vi "EstimateTargetingInformation.vi"(0 "X (in) [t0]":dbl, 5 "Y (in) [t0]":dbl, 7 "Robot Heading (deg)":dbl, 12 "Acceptable Heading Error (deg)":dbl, 13 "Min Timed Aligned (ms)":u32) -> (4 "Pointed At Target":bool, 6 "Heading to Target (deg)":dbl, 8 "Distance to Target (in)":dbl, 15 "Targeting Information":dbl[](array[numeric]))   [LabVIEW 2020]
doc: "This VI estimates the robot's heading and distance to the nearest requested scoring location."
uses:
  <vilib>/Rock Robotics/WPI/DriverStation/WPI_DriverStationAllianceInfo.ctl
  GlobalArm.vi
  GlobalDriverStationData.vi
  GlobalPoseAndTargeting.vi
  GlobalDriverStationCommands.vi
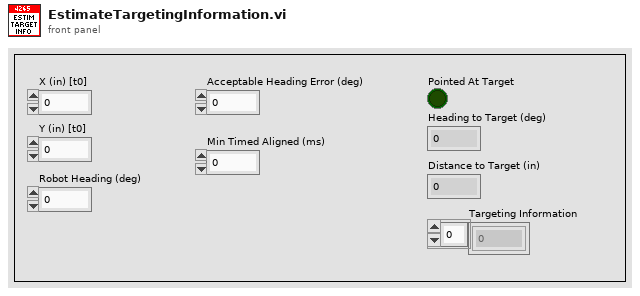
[diagram p1: front panel]
types:
  T1 = typedef "WPI_DriverStationAllianceInfo.ctl" = enum16{"Red", "Blue", "Invalid"}
  T2 = enum16{"Low Cube", "Mid Cube", "High Cube", "Low Cone", "Mid Cone", "High Cone"}
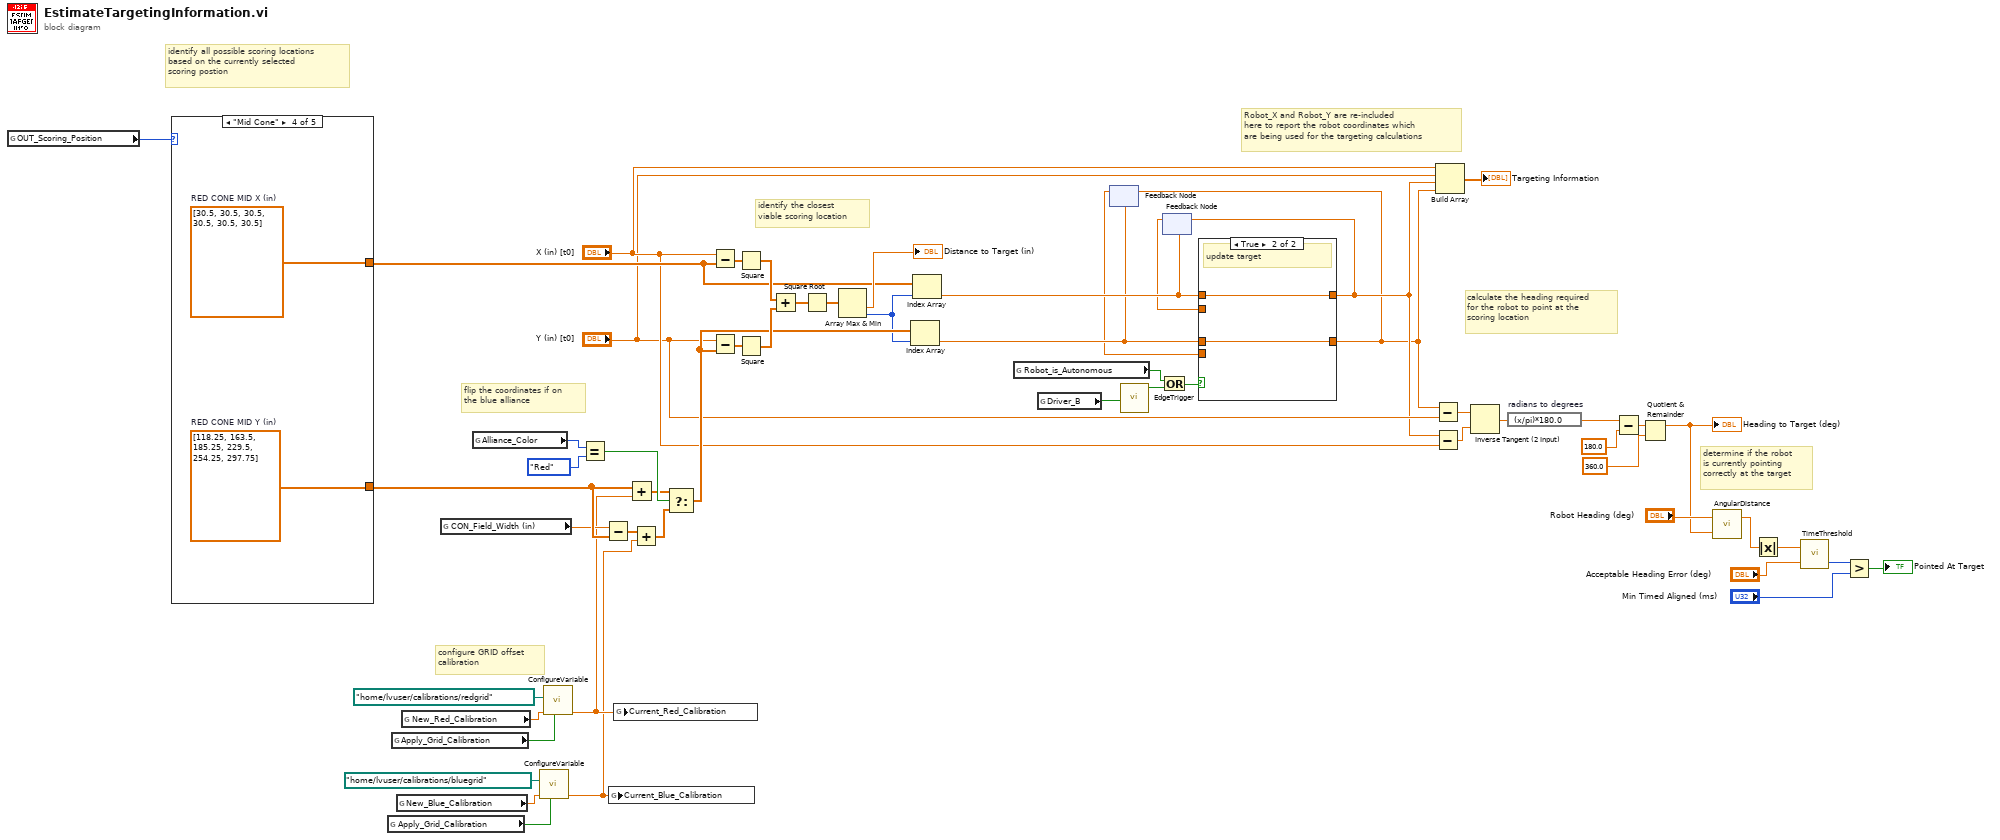
[diagram p0: block diagram]
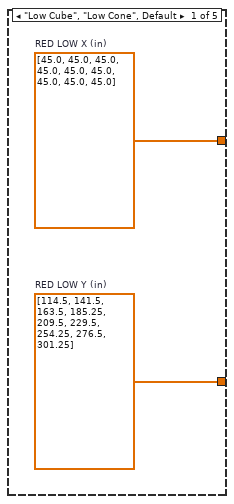
[diagram p3: hidden frame]
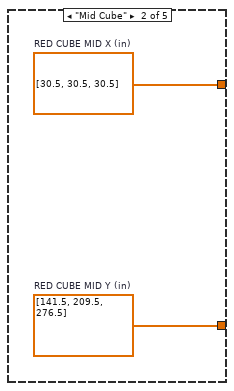
[diagram p4: hidden frame]
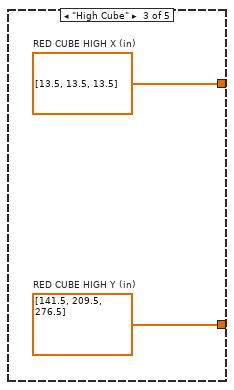
[diagram p5: hidden frame]
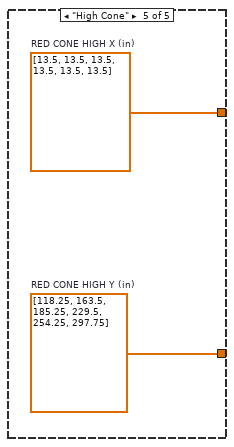
[diagram p6: hidden frame]
diagram:
  # "configure GRID offset\ncalibration"
  # "Robot_X and Robot_Y are re-included\nhere to report the robot coordinates which\nare being used for the targeting calculations"
  # "determine if the robot\nis currently pointing\ncorrectly at the target"
  # "calculate the heading required\nfor the robot to point at the\nscoring location"
  # "identify the closest\nviable scoring location"
  # "flip the coordinates if on\nthe blue alliance"
  # "identify all possible scoring locations\nbased on the currently selected\nscoring postion"
  n1 = global read "GlobalArm.vi" "OUT_Scoring_Position"() -> (w13:T2)
  n2 = case shown="\"Mid Cone\"" w13 {
    tunnel: [w57 w59 w61 w63 w65] -> w41
    tunnel: [w56 w58 w60 w62 w64] -> w51
    frame "Low Cube", "Low Cone", Default {
      w56 = dbl[] [114.5, 141.5, 163.5, 185.25, 209.5, 229.5, 254.25, 276.5, 301.25]  # RED LOW Y (in)
      w57 = dbl[] [45.0, 45.0, 45.0, 45.0, 45.0, 45.0, 45.0, 45.0, 45.0]  # RED LOW X (in)
    }
    frame "Mid Cube" {
      w58 = dbl[] [141.5, 209.5, 276.5]  # RED CUBE MID Y (in)
      w59 = dbl[] [30.5, 30.5, 30.5]  # RED CUBE MID X (in)
    }
    frame "High Cube" {
      w60 = dbl[] [141.5, 209.5, 276.5]  # RED CUBE HIGH Y (in)
      w61 = dbl[] [13.5, 13.5, 13.5]  # RED CUBE HIGH X (in)
    }
    frame "Mid Cone" {
      w62 = dbl[] [118.25, 163.5, 185.25, 229.5, 254.25, 297.75]  # RED CONE MID Y (in)
      w63 = dbl[] [30.5, 30.5, 30.5, 30.5, 30.5, 30.5]  # RED CONE MID X (in)
    }
    frame "High Cone" {
      w64 = dbl[] [118.25, 163.5, 185.25, 229.5, 254.25, 297.75]  # RED CONE HIGH Y (in)
      w65 = dbl[] [13.5, 13.5, 13.5, 13.5, 13.5, 13.5]  # RED CONE HIGH X (in)
    }
  }
  n3 = global read "GlobalPoseAndTargeting.vi" "Apply_Grid_Calibration"() -> (w5:bool)
  n4 = global read "GlobalPoseAndTargeting.vi" "Apply_Grid_Calibration"() -> (w9:bool)
  n5 = global read "GlobalPoseAndTargeting.vi" "New_Blue_Calibration"() -> (w6:dbl)
  n6 = global read "GlobalPoseAndTargeting.vi" "New_Red_Calibration"() -> (w10:dbl)
  n7 = global read "GlobalPoseAndTargeting.vi" "CON_Field_Width (in)"() -> (w49:dbl)
  n8 = global read "GlobalDriverStationData.vi" "Alliance_Color"() -> (w54:T1)
  n9 = call "ConfigureVariable.vi"("Apply New Setpoint"=w5, "New Setpoint Value"=w6, "Setpoint Save Location"=path "/home/lvuser/calibrations/bluegrid") -> ("Selected Setpoint Value"=w4:dbl)  [unwired: 8 in]
  n10 = call "ConfigureVariable.vi"("Apply New Setpoint"=w9, "New Setpoint Value"=w10, "Setpoint Save Location"=path "/home/lvuser/calibrations/redgrid") -> ("Selected Setpoint Value"=w8:dbl)  [unwired: 8 in]
  n11 = Equal?(x=w54, y=WPI_DriverStationAllianceInfo."Red") -> (x = y?=w52:bool)
  n12 = Subtract(x=w49, y=w51) -> (x-y=w50:dbl[])
  n13 = global write "GlobalPoseAndTargeting.vi" "Current_Blue_Calibration"(w4) -> ()
  n14 = global write "GlobalPoseAndTargeting.vi" "Current_Red_Calibration"(w8) -> ()
  n15 = Add(x=w51, y=w8) -> (x+y=w20:dbl[])
  n16 = Add(x=w50, y=w4) -> (x+y=w21:dbl[])
  n17 = Select(t=w20, s=w52, f=w21) -> (s? t:f=w40:dbl[])
  n18 = Subtract(x="X (in) [t0]", y=w41) -> (x-y=w48:dbl[])
  n19 = Subtract(x="Y (in) [t0]", y=w40) -> (x-y=w47:dbl[])
  n20 = Square(x=w48) -> (x^2=w46:dbl[])
  n21 = Square(x=w47) -> (x^2=w45:dbl[])
  n22 = Add(x=w46, y=w45) -> (x+y=w44:dbl[])
  n23 = Square Root(x=w44) -> (sqrt(x)=w43:dbl[])
  n24 = Array Max & Min(array=w43) -> (min value=→"Distance to Target (in)":dbl, min index (indices)=w39:i32)  [unwired: 2 out]
  n25 = Index Array(array=w40, index=w39) -> (element=w16:dbl)
  n26 = Index Array(array=w41, index=w39) -> (element=w18:dbl)
  n27 = global read "GlobalDriverStationData.vi" "Robot_is_Autonomous"() -> (w1:bool)
  n28 = global read "GlobalDriverStationCommands.vi" "Driver_B"() -> (w12:bool)
  n29 = feedback #1(w16) -> (w14:dbl)
  n30 = call "EdgeTrigger.vi"("Input Signal"=w12) -> ("Rising Edge Trigger"=w2:bool)  [unwired: 2 out]
  n31 = Or(x=w1, y=w2) -> (x .or. y?=w3:bool)
  n32 = feedback #2(w18) -> (w17:dbl)
  n33 = case shown="True" w3 {
    tunnel: w18 -> [_ w69]
    tunnel: w16 -> [_ w68]
    tunnel: [w67 w69] -> w19
    tunnel: [w66 w68] -> w15
    tunnel: w17 -> [w67 _]
    tunnel: w14 -> [w66 _]
    frame False {
      # "use latched target"
    }
    frame True {
      # "update target"
    }
  }
  n34 = feedback-in #1(w15) -> ()
  n35 = feedback-in #2(w19) -> ()
  n36 = Subtract(x=w15, y="Y (in) [t0]") -> (x-y=w37:dbl)
  n37 = Subtract(x=w19, y="X (in) [t0]") -> (x-y=w36:dbl)
  n38 = Build Array("X (in) [t0]", "Y (in) [t0]", w19, w15) -> (→"Targeting Information":dbl[])
  n39 = Inverse Tangent (2 Input)(1:w36, 2:w37) -> (0:w38:dbl)
  n40 = expression code="(x/pi)*180.0" "radians to degrees"(w38) -> (w25:dbl)
  n41 = Subtract(x=w25, y=180.0) -> (x-y=w24:dbl)
  n42 = Quotient & Remainder(x=w24, y=360.0) -> (x-y*floor(x/y)=w22:dbl)  [unwired: 1 out]
  "Heading to Target (deg)" <- w22
  n43 = call "AngularDistance.vi"("Goal Angle (deg) [0,360]"=w22, "Current Angle (deg) [-Inf,+Inf]"="Robot Heading (deg)") -> ("Signed Angular Distance (deg) [-180,+180]"=w32:dbl)  [unwired: 1 out]
  n44 = Absolute Value(x=w32) -> (abs(x)=w30:dbl)
  n45 = call "TimeThreshold.vi"("Threshold"="Acceptable Heading Error (deg)", "Current Value"=w30) -> ("Time Below Threshold (ms)"=w29:u32)  [unwired: 1 out]
  n46 = Greater?(x=w29, y="Min Timed Aligned (ms)") -> (0:→"Pointed At Target":bool)
